vi "WFS Get Spotfield Image Copy.vi"(8 "error in (no error)":errorcluster {"code" format="%.0x"}, 11 "instrument handle":refnum<visa-resource-name>) -> (0 "error out":errorcluster {"code" format="%.0x"}, 1 "Rows":i32, 2 "ImageBuf":u8[](array[numeric]), 3 "instrument handle out":refnum<visa-resource-name>, 4 "Columns":i32)   [LabVIEW 2020]
doc: "This VI returns a copy of the spotfield image taken by VIs TakeSpotfieldImage() or TakeSpotfieldImageAutoExpos() into the user provided buffer ImageBuf.\nIt returns also the image size.\n\nNote: This VI is not available in Highspeed Mode!"
uses:
  WFS_32.dll
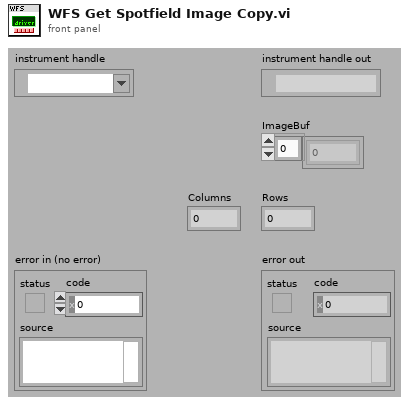
[diagram p1: front panel]
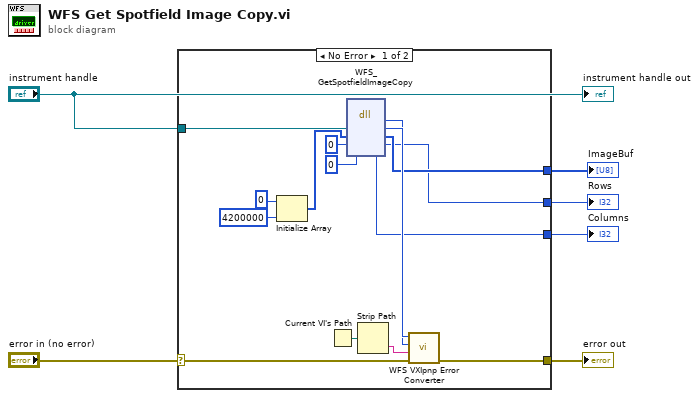
[diagram p0: block diagram]
diagram:
  n1 = case shown="No Error" "error in (no error)" {
    selector: "error in (no error)" -> [w16 w22]
    tunnel: [w15 w22] -> w6
    tunnel: "instrument handle" -> [w20 _]
    tunnel: [w11 _] -> w3
    tunnel: [w9 _] -> w2
    tunnel: [w7 _] -> w1
    frame No Error {
      n2 = Initialize Array(u8 0 ("element"), 4200000 ("dimension size")) -> (w14:u8[])
      n3 = Current VI's Path() -> (path=w21:path)
      n4 = dll-call lib="WFS_*.*" fn="WFS_GetSpotfieldImageCopy"("Instrument Handle"=w20, "ImageBuf"=w14, "Rows"=0, "Columns"=0) -> (w18:i32, "Instrument Handle"=w19:u32, "ImageBuf"=w11:u8[], "Rows"=w9:i32, "Columns"=w7:i32)  [unwired: 3 in, 2 out]
      n5 = Strip Path(path=w21) -> (name=w17:string)  [unwired: 1 out]
      n6 = call "WFS VXIpnp Error Converter.vi"("error in (no error)"=w16, "Name Of VI (\"\")"=w17, "CVI Error Code (0)"=w18, "instrument handle"=w19) -> ("error out"=w15:errorcluster)  [unwired: 6 in, 1 out]
    }
    frame Error {
    }
  }
  "error out" <- w6
  "ImageBuf" <- w3
  "Rows" <- w2
  "Columns" <- w1
  "instrument handle out" <- "instrument handle"
